vi "Remove_All_Escaped.vi"(0 "Input String":string) -> (1 "Output String":string, 2 "Chars Removed":i32)   [LabVIEW 2011]
doc: "This VI removes all escape sequences from the input string. The escape character is the backslash."
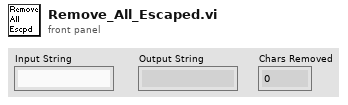
[diagram p1: front panel]
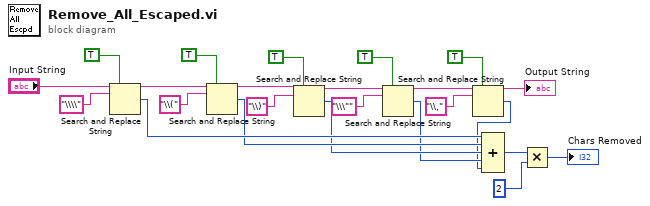
[diagram p0: block diagram]
diagram:
  n1 = Search and Replace String(replace all?=TRUE ("replace all? (F)"), input string="Input String", search string="\\\\") -> (result string=w20:string, number of replacements=w8:i32)  [unwired: 5 in, 2 out]
  n2 = Search and Replace String(replace all?=TRUE ("replace all? (F)"), input string=w20, search string="\\(") -> (result string=w17:string, number of replacements=w7:i32)  [unwired: 5 in, 2 out]
  n3 = Search and Replace String(replace all?=TRUE ("replace all? (F)"), input string=w17, search string="\\)") -> (result string=w14:string, number of replacements=w6:i32)  [unwired: 5 in, 2 out]
  n4 = Search and Replace String(replace all?=TRUE ("replace all? (F)"), input string=w14, search string="\\\"") -> (result string=w11:string, number of replacements=w5:i32)  [unwired: 5 in, 2 out]
  n5 = Search and Replace String(replace all?=TRUE ("replace all? (F)"), input string=w11, search string="\\,") -> (result string=→"Output String":string, number of replacements=w4:i32)  [unwired: 5 in, 2 out]
  n6 = Compound Arithmetic op=ADD(w8, w7, w6, w5, w4) -> (w3:i32)
  n7 = Multiply(x=w3, y=2) -> (x*y=→"Chars Removed":i32)
